vi "RvsTemp_Lakeshore_crh.vi"() -> ()   [LabVIEW 2017]
uses:
  sub_vis/ke26xx/Public/Channel.ctl
  sub_vis/ke26xx/KE26XX.lvlib
panel:
  in  "Units":i8(ring)=1 items=["Ohms"=1, "m-Ohms (1e-3)"=2, "u-Ohms (1e-6)"=3, ""=0]
  out "Neg. V (V)":dbl=1.0 format="%.;%#_g"
  out "Neg. I (A)":dbl=1.0 format="%.;%#_g"
  out "Pos. V (V)":dbl=1.0 format="%.;%#_g"
  out "Pos. I (A)":dbl=1.0 format="%.;%#_g"
  out "Node Out":string
  in  "Plot Scales":u16(ring) items=["Autoscale All", "Autoscale X", "Autoscale Y", "Manual Scale"]
  in  "Control Temp":bool=TRUE
  in  "Update":bool caption="Boolean"
  in  "Tab Control":enum32{"Configure", "Heater", "Auto"}(tab)
  in  "Curve Number (0)":dbl min=0.0 max=41.0 step=1.0
  in  "Sensor Type (0: Silicon Diode)":i8(ring) items=["Silicon Diode", "GaAIAS Diode", "100 Ohm Platinum/250", "100 Ohm Platinum/500", "1000 Ohm Platinum", "NTC RTD", "Thermo/25mV", "Thermo/50mV"]
  in  "Heater Range (0: Off)":u16(ring) items=["Off", "Low (0.5W)", "Med (5W)", "High (50W)"]
  in  "Manual Output (%)":dbl min=0.0 max=100.0 step=0.001 format="%.;%.3f"
  out "Heater Output":dbl(slide) scale=0.0..100.0
  in  "Loop (0: 1)":u16(ring) items=["1", "2"]
  in  "Rate (D)":dbl min=0.0 max=1000.0 step=0.1 format="%.;%.1f"
  in  "Reset (I)":dbl min=0.0 max=1000.0 step=0.1 format="%.;%.1f"
  in  "Gain (P)":dbl min=0.0 max=1000.0 step=0.1 format="%.;%.1f"
  in  "Ramp Rate\n(K/min)":dbl=0.1 min=0.0 max=100.0 step=0.1 format="%.1f"
  in  "Ramping \nOn/Off (F: Off)":bool
  in  "Setpoint (K)":dbl min=0.0 max=1000.0 step=0.1 format="%.;%.1f"
  in  "Control Mode (0: Manual PID)":u16(ring) items=["Manual PID", "Zone", "Open Loop", "AutoTune PID", "AutoTune PI", "AutoTune P"]
  out "temp vs time":cluster{"Y":dbl[], "Y":dbl[]}[](graph)
  out "Current (mA):":dbl=19.983 format="%.;%.4f"
  out "Voltage (mV):":dbl=19.983 format="%.;%.4f"
  in  "Limit (mA)":dbl=1.0 format="%.;%#_g"
  in  "Level (mV)":dbl=1.0 format="%.;%#_g"
  in  "Channel (A):":T1
  in  "VISA resource name":refnum<visa-resource-name>
  in  "Comments":string="comments here"
  in  "Y Max.":dbl min=0.0 max=1000.0 step=0.1 format="%.;%.1f"
  in  "Y Min.":dbl min=0.0 max=1000.0 step=0.1 format="%.;%.1f"
  in  "X Max.":dbl min=0.0 max=1000.0 step=0.1 format="%.;%.1f"
  in  "X Min.":dbl min=0.0 max=1000.0 step=0.1 format="%.;%.1f"
  in  "Reset":bool
  out "Resistance":dbl=19.983 format="%.;%_5f"
  in  "Log R":bool
  in  "Filename 2":string="07_YBCO_EOS_20K_outofplane_pumpon_5ps_"
  in  "Extension":string=".dat"
  in  "Filename":string="filename"
  in  "Path":string="C:\\path\\to\\data"
  in  "Save":bool caption="Boolean"
  in  "Log Temp":bool=TRUE
  in  "Lakeshore VISA session":refnum<visa-resource-name>="COM1"
  in  "Lakeshore Input (0: A)":u16(ring)=2 items=["A", "B", "ITC5035"]
  out "Temperature (K)":dbl=19.983 format="%.2f"
  in  "Stop":bool
  out "R vs T":cluster{"Y":dbl[], "Y":dbl[]}[](graph)
  # "Temperature Sensor"
  # "Set Filename and Path"
  # "Heater Control"
  # "Resistance Measurement"
  # "Written by Cassi Hunt, November 2012\n\nTemperature Control: LakeShore 331\nSourceMeter: Keithley 2635A"
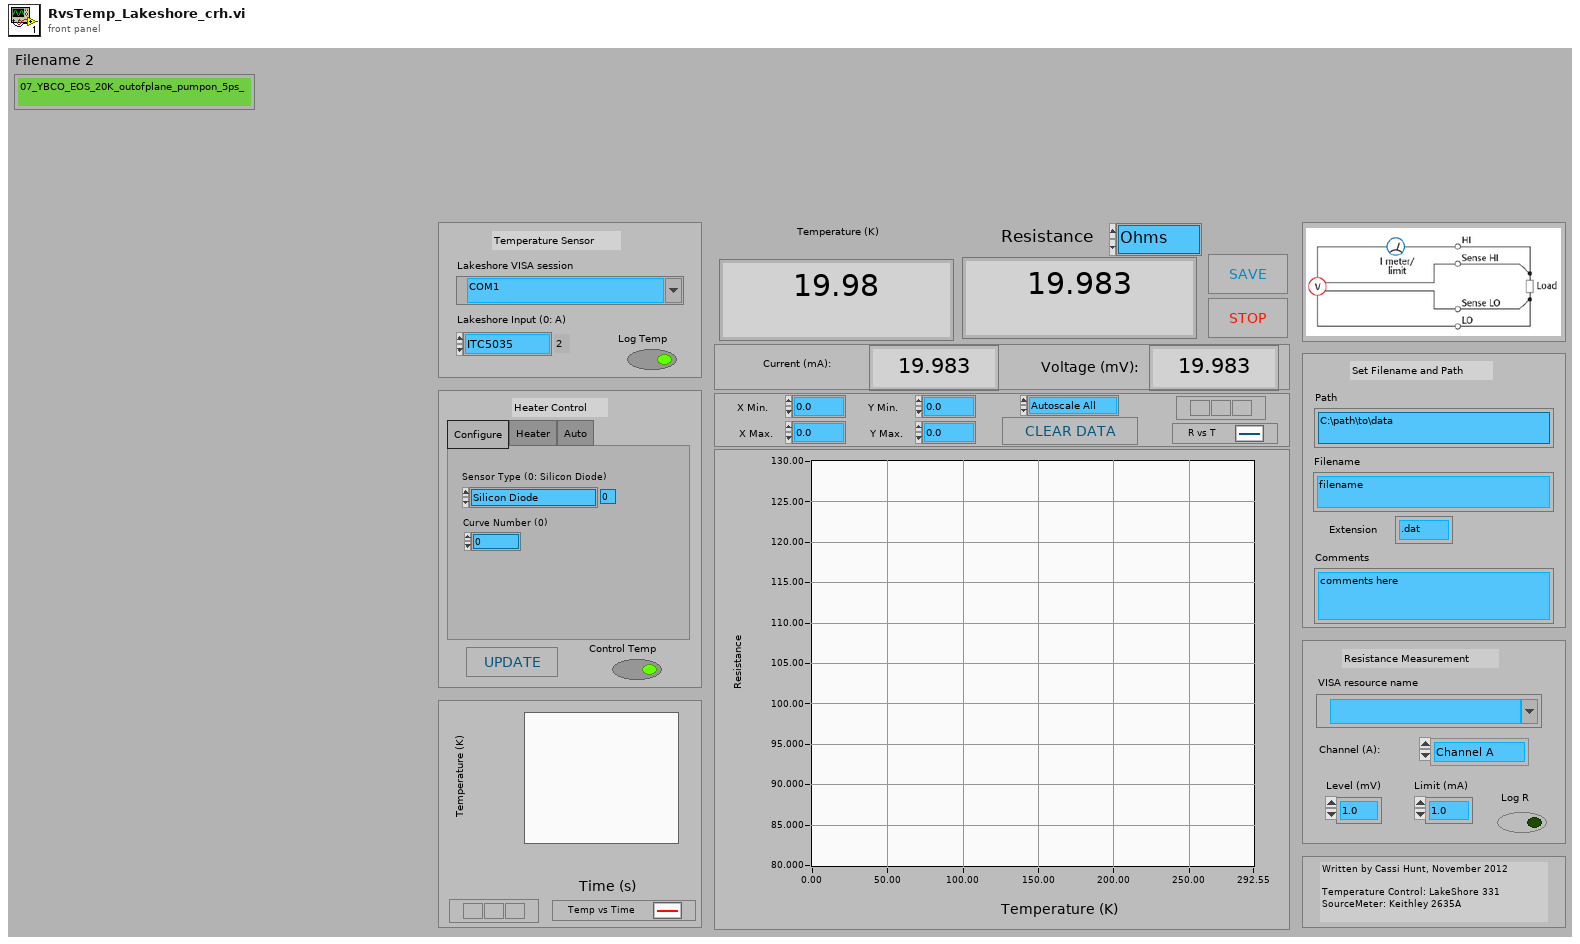
[diagram p1: front panel]
types:
  T1 = typedef "KE26XX.lvlib/Channel.ctl" = enum32{"Channel A", "Channel B"}
  T2 = enum32{"Current", "Voltage", "IV", "Resistance", "Power"}
  T3 = typedef "ke26xx.lvlib/Channel.ctl" = enum32{"Channel A", "Channel B"}
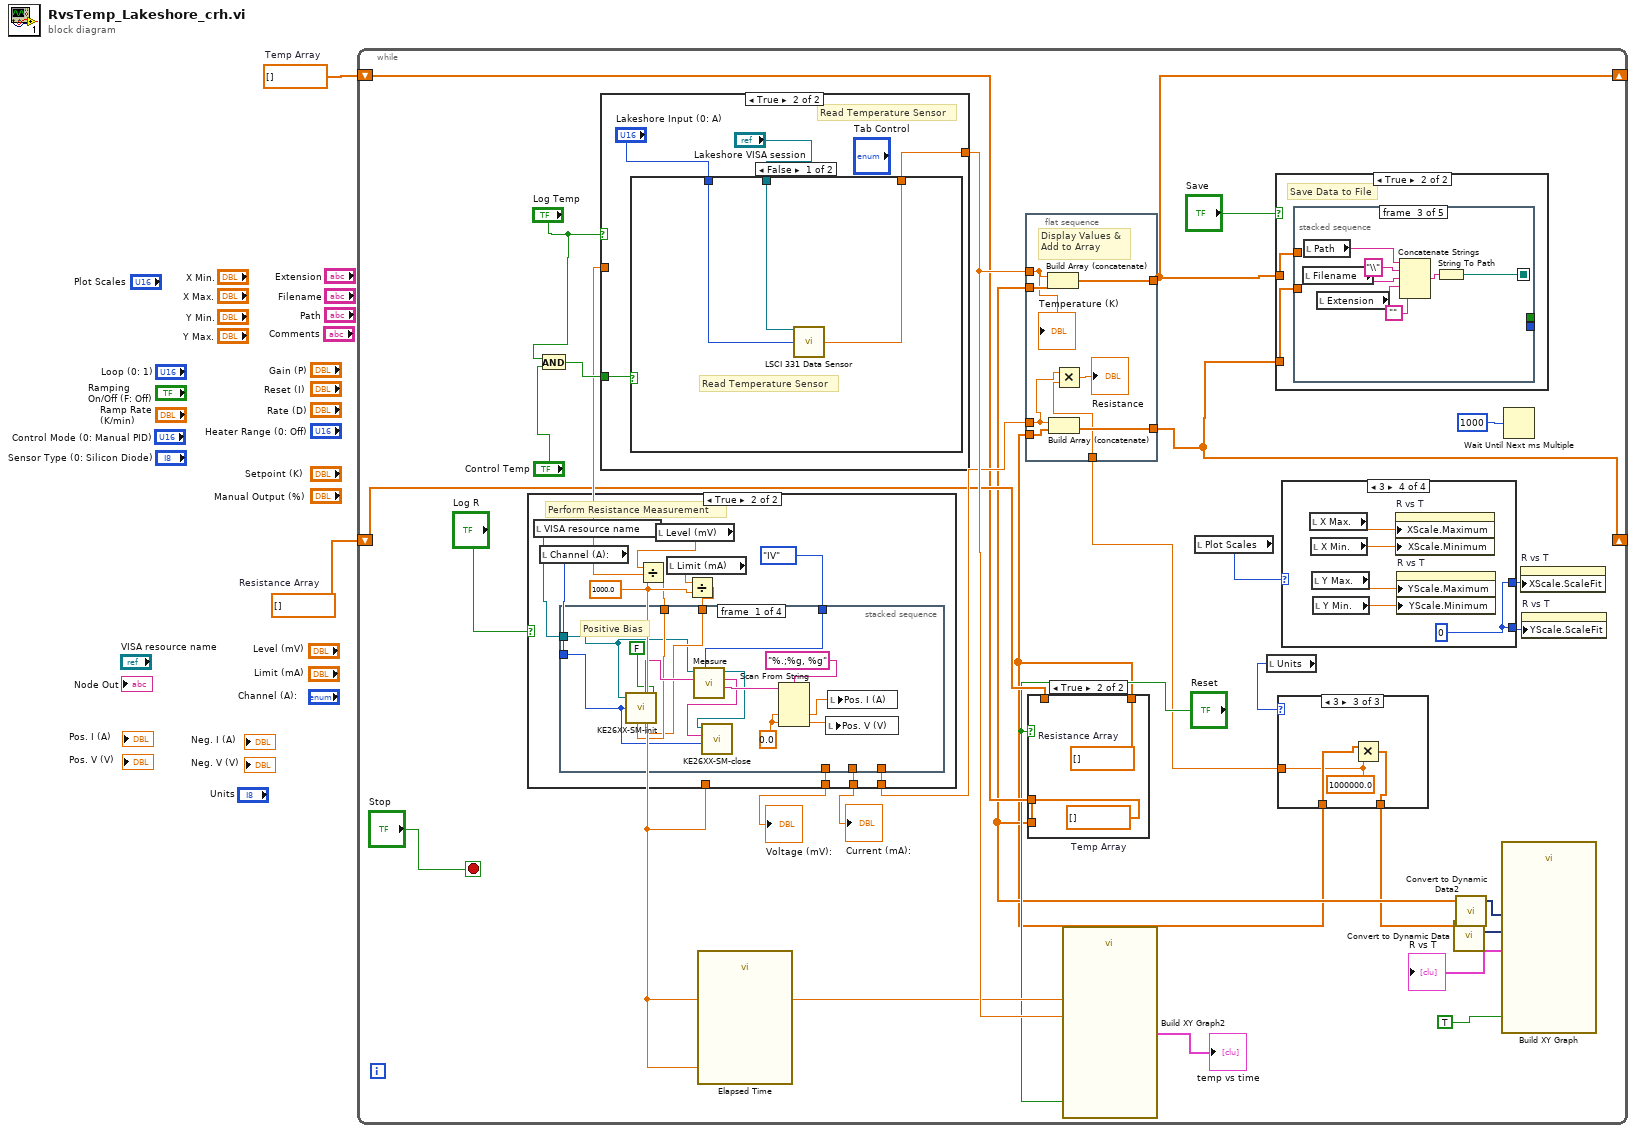
[diagram p0: block diagram]
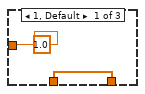
[diagram p2: hidden frame]
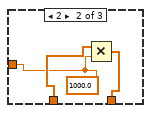
[diagram p3: hidden frame]
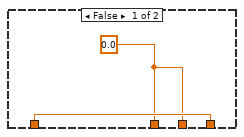
[diagram p5: hidden frame]
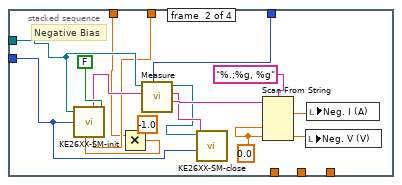
[diagram p6: hidden frame]
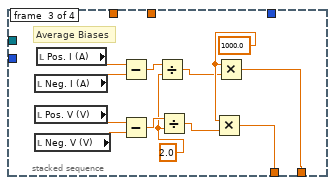
[diagram p7: hidden frame]
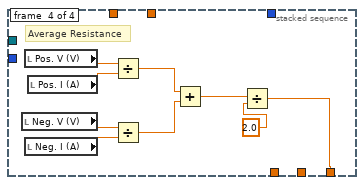
[diagram p8: hidden frame]
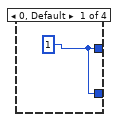
[diagram p9: hidden frame]
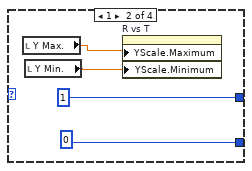
[diagram p10: hidden frame]
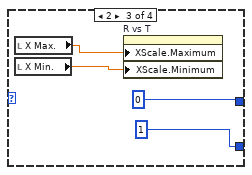
[diagram p11: hidden frame]
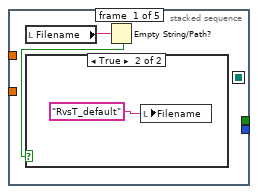
[diagram p13: hidden frame]
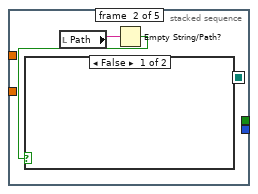
[diagram p15: hidden frame]
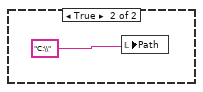
[diagram p16: hidden frame]
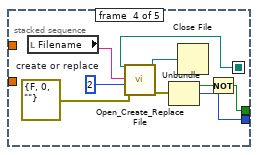
[diagram p17: hidden frame]
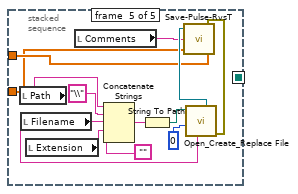
[diagram p18: hidden frame]
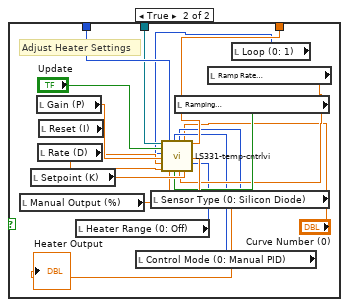
[diagram p20: hidden frame]
diagram:
  w1 = dbl[] []  # Resistance Array
  w2 = dbl[] []  # Temp Array
  n1 = while {
    shift-right: [w24] -> _
    shift-left: w2 -> [w13]
    shift-right: [w5] -> _
    shift-left: w1 -> [w14]
    stop <- "Stop" stop-if-true
    n2 = And(x="Log Temp", y="Control Temp") -> (x .and. y?=w27:bool)
    n3 = call "Elapsed Time"() -> ("Elapsed Time (s)"=w16:dbl)  [unwired: 12 in, 7 out]
    n4 = case shown="True" "Log R" {
      tunnel: [w46 w49] -> w19
      tunnel: [w45 w48] -> w18
      tunnel: [w45 w47] -> w17
      tunnel: w16 -> [w46 _]
      frame False {
        w45 = 0.0
      }
      frame True {
        w54 = 1000.0
        # "Perform Resistance Measurement"
        n5 = local read "VISA resource name"() -> (w57:refnum<visa-resource-name>)
        n6 = local read "Channel (A):"() -> (w56:T3)
        n7 = local read "Level (mV)"() -> (w51:dbl)
        n8 = Divide(x=w51, y=w54) -> (x/y=w50:dbl)
        n9 = local read "Limit (mA)"() -> (w53:dbl)
        n10 = Divide(x=w53, y=w54) -> (x/y=w52:dbl)
        n11 = stacked-sequence {
          tunnel: w57 -> [w64 w83 _ _]
          tunnel: w56 -> [w58 w73 _ _]
          tunnel: T2."IV" ("Measure Function (Current)") -> [w67 w81 _ _]
          tunnel: w52 -> [w65 w82 _ _]
          tunnel: w50 -> [w66 w76 _ _]
          tunnel: [_ _ _ w100] -> w49
          tunnel: [_ _ w89 _] -> w48
          tunnel: [_ _ w88 _] -> w47
          frame #0 {
            w70 = 0.0
            # "Positive Bias"
            n12 = call "KE26XX-SM-init.vi"("VISA resource name"=w64, "Channel (Channel A)"=w58, "Level"=w66, "Error Query (False)"=FALSE, "Limit"=w65) -> ("Node Out"=w68:string)  [unwired: 3 in, 1 out]
            n13 = call "Measure.vi"("Function (Current)"=w67, "Node In"=w68, "VISA resource name"=w64) -> ("Output"=w69:string, "Node Out"=w59:string, "VISA resource name out"=w60:refnum<visa-resource-name>)  [unwired: 4 in, 2 out]
            n14 = call "KE26XX-SM-close.vi"("Channel (Channel A)"=w58, "Node In"=w59, "VISA resource name"=w60) -> ()  [unwired: 8 in, 1 out]
            n15 = Scan From String(format string="%.;%g, %g", input string=w69, default 1=w70, default 2=w70) -> (output 1=w62:dbl, output 2=w61:dbl)  [unwired: 2 in, 3 out]
            n16 = local write "Pos. V (V)"(w61) -> ()
            n17 = local write "Pos. I (A)"(w62) -> ()
          }
          frame #1 {
            w84 = 0.0
            # "Negative Bias"
            n18 = Multiply(x=w76, y=-1.0) -> (x*y=w75:dbl)
            n19 = call "KE26XX-SM-init.vi"("VISA resource name"=w83, "Channel (Channel A)"=w73, "Level"=w75, "Error Query (False)"=FALSE, "Limit"=w82) -> ("Node Out"=w86:string)  [unwired: 3 in, 1 out]
            n20 = call "Measure.vi"("Function (Current)"=w81, "Node In"=w86, "VISA resource name"=w83) -> ("Output"=w85:string, "Node Out"=w74:string, "VISA resource name out"=w72:refnum<visa-resource-name>)  [unwired: 4 in, 2 out]
            n21 = call "KE26XX-SM-close.vi"("Channel (Channel A)"=w73, "Node In"=w74, "VISA resource name"=w72) -> ()  [unwired: 8 in, 1 out]
            n22 = Scan From String(format string="%.;%g, %g", input string=w85, default 1=w84, default 2=w84) -> (output 1=w79:dbl, output 2=w78:dbl)  [unwired: 2 in, 3 out]
            n23 = local write "Neg. V (V)"(w78) -> ()
            n24 = local write "Neg. I (A)"(w79) -> ()
          }
          frame #2 {
            w93 = 2.0
            w92 = 1000.0
            # "Average Biases"
            n25 = local read "Neg. I (A)"() -> (w98:dbl)
            n26 = local read "Pos. V (V)"() -> (w97:dbl)
            n27 = local read "Neg. V (V)"() -> (w96:dbl)
            n28 = local read "Pos. I (A)"() -> (w99:dbl)
            n29 = Subtract(x=w99, y=w98) -> (x-y=w94:dbl)
            n30 = Subtract(x=w97, y=w96) -> (x-y=w95:dbl)
            n31 = Divide(x=w94, y=w93) -> (x/y=w91:dbl)
            n32 = Divide(x=w95, y=w93) -> (x/y=w90:dbl)
            n33 = Multiply(x=w92, y=w90) -> (x*y=w88:dbl)
            n34 = Multiply(x=w92, y=w91) -> (x*y=w89:dbl)
          }
          frame #3 {
            # "Average Resistance"
            n35 = local read "Neg. V (V)"() -> (w106:dbl)
            n36 = local read "Pos. V (V)"() -> (w108:dbl)
            n37 = local read "Neg. I (A)"() -> (w105:dbl)
            n38 = local read "Pos. I (A)"() -> (w107:dbl)
            n39 = Divide(x=w108, y=w107) -> (x/y=w104:dbl)
            n40 = Divide(x=w106, y=w105) -> (x/y=w103:dbl)
            n41 = Add(x=w104, y=w103) -> (x+y=w102:dbl)
            n42 = Divide(x=w102, y=2.0) -> (x/y=w100:dbl)
          }
        }
      }
    }
    "Voltage (mV):" <- w17
    "Current (mA):" <- w18
    n43 = case shown="True" "Log Temp" {
      tunnel: [w168 w169] -> w25
      tunnel: w16 -> [w168 _]
      tunnel: w27 -> [_ w172]
      frame False {
      }
      frame True {
        # "Read Temperature Sensor"
        n44 = case shown="False" w172 {
          tunnel: "Lakeshore Input (0: A)" -> [w173 w192]
          tunnel: "Lakeshore VISA session" -> [w174 w191]
          tunnel: [w175 w183] -> w169
          frame False {
            # "Read Temperature Sensor"
            n45 = call "LSCI 331 Data Sensor.vi"("VISA session"=w174, "Input (0: A)"=w173) -> ("Kelvin Reading"=w175:dbl)  [unwired: 1 in, 12 out]
          }
          frame True {
            # "Adjust Heater Settings"
            n46 = local read "Manual Output (%)"() -> (w185:dbl)
            n47 = local read "Setpoint (K)"() -> (w186:dbl)
            n48 = local read "Gain (P)"() -> (w189:dbl)
            n49 = local read "Rate (D)"() -> (w187:dbl)
            n50 = local read "Reset (I)"() -> (w188:dbl)
            n51 = local read "Heater Range (0: Off)"() -> (w179:u16)
            n52 = local read "Control Mode (0: Manual PID)"() -> (w178:u16)
            n53 = local read "Sensor Type (0: Silicon Diode)"() -> (w177:i8)
            n54 = local read "Ramping \nOn/Off (F: Off)"() -> (w182:bool)
            n55 = local read "Ramp Rate\n(K/min)"() -> (w180:dbl)
            n56 = local read "Loop (0: 1)"() -> (w181:u16)
            n57 = call "LS331-temp-cntrlvi.vi"("VISA resource name"=w191, "Configure (False)"="Update", "Loop (0: 1)"=w181, "Gain (P) (0.0)"=w189, "Reset (I) (0.0)"=w188, "Rate (D) (0)"=w187, "Input (0: A)"=w192, "Control Mode (0: Manual PID)"=w178, "Ramping On/Off (F: Off)"=w182, "Sensor Type (0: Silicon Diode)"=w177, "Rate Value (0.1)"=w180, "Curve Number (0)"="Curve Number (0)", "Setpoint (0.0000)"=w186, "Manual Output (0.000)"=w185, "Heater Range (0: Off)"=w179) -> ("Loop 1\nHeater Output"=→"Heater Output":dbl, "Kelvin Reading"=w183:dbl)  [unwired: 1 in, 2 out]
          }
        }
      }
    }
    n58 = flat-sequence {
      tunnel: w9 -> [w129]
      tunnel: [w130] -> w24
      tunnel: w25 -> [w126]
      tunnel: w19 -> [w125]
      tunnel: w7 -> [w127]
      tunnel: [w128] -> w5
      tunnel: w4 -> [w123]
      frame #0 {
        # "Display Values &\nAdd to Array"
        n59 = Build Array (concatenate)(w126, w129) -> (w130:dbl[])
        n60 = Build Array (concatenate)(w125, w127) -> (w128:dbl[])
        n61 = Multiply(x=w125, y=w123) -> (x*y=→"Resistance":dbl)
        "Temperature (K)" <- w126
      }
    }
    n62 = case shown="True" "Reset" {
      tunnel: [w42 w44] -> w7
      tunnel: w14 -> [w42 _]
      tunnel: [w41 w43] -> w9
      tunnel: w13 -> [w41 _]
      frame False {
      }
      frame True {
        w43 = dbl[] []  # Temp Array
        w44 = dbl[] []  # Resistance Array
      }
    }
    n63 = call "Build XY Graph2"("Reset"="Reset", "Y Input"=w25, "X Input"=w16) -> ("XY Graph"=→"temp vs time":cluster{"Y":dbl[], "Y":dbl[]}[])  [unwired: 2 in, 6 out]
    n64 = local read "Plot Scales"() -> (w23:u16)
    n65 = local read "Units"() -> (w11:i8)
    n66 = case shown="True" "Save" {
      tunnel: w24 -> [_ w132]
      tunnel: w5 -> [_ w131]
      frame False {
      }
      frame True {
        # "Save Data to File"
        n67 = stacked-sequence {
          seq-local: [_ _ w143 _ _] -> [_ _ _ w148 _]
          tunnel: [_ _ _ w149 _] -> _
          tunnel: [_ _ _ w147 _] -> _
          tunnel: w132 -> [_ _ _ _ w157]
          tunnel: w131 -> [_ _ _ _ w156]
          frame #0 {
            n68 = local read "Filename"() -> (w134:string)
            n69 = Empty String/Path?(string/path=w134) -> (empty?=w133:bool)
            n70 = case shown="True" w133 {
              frame False {
              }
              frame True {
                n71 = local write "Filename"("RvsT_default") -> ()
              }
            }
          }
          frame #1 {
            n72 = local read "Path"() -> (w137:string)
            n73 = Empty String/Path?(string/path=w137) -> (empty?=w136:bool)
            n74 = case shown="False" w136 {
              frame False {
              }
              frame True {
                n75 = local write "Path"("C:\\") -> ()
              }
            }
          }
          frame #2 {
            n76 = local read "Filename"() -> (w139:string)
            n77 = local read "Path"() -> (w142:string)
            n78 = local read "Extension"() -> (w140:string)
            n79 = Concatenate Strings(w142, "\\" ("Substring"), w139, w140, "") -> (w144:string)
            n80 = String To Path(string=w144) -> (path=w143:path)
          }
          frame #3 {
            w151 = i16 2  # create or replace
            n81 = local read "Filename"() -> (w146:string)
            n82 = call <vilib>:"Open_Create_Replace File.vi"("default name"=w146, "error in (no error)"=errorcluster {"status"=FALSE, "code"=0, "source"=""}, "function (open:0)"=w151, "file path"=w148) -> ("error out"=w153:errorcluster, "refnum"=w152:refnum<file>)  [unwired: 2 in, 4 out]
            n83 = Unbundle(w153) -> ("status"=w150:bool, "code"=w147:i32)  [unwired: 1 out]
            n84 = Close File(refnum=w152) -> ()  [unwired: 1 in, 2 out]
            n85 = Not(x=w150) -> (.not. x?=w149:bool)
          }
          frame #4 {
            n86 = local read "Path"() -> (w158:string)
            n87 = local read "Filename"() -> (w164:string)
            n88 = local read "Extension"() -> (w160:string)
            n89 = local read "Comments"() -> (w155:string)
            n90 = Concatenate Strings(w158, "\\" ("Substring"), w164, w160, "") -> (w161:string)
            n91 = String To Path(string=w161) -> (path=w162:path)
            n92 = call <vilib>:"Open_Create_Replace File.vi"("default name"=w164, "function (open:0)"=i16 0 ("create or replace"), "file path"=w162) -> ("error out"=w166:errorcluster, "refnum"=w167:refnum<file>)  [unwired: 3 in, 4 out]
            n93 = call "Save-Pulse-RvsT.vi"("X-Values"=w157, "error in"=w166, "Y-Values"=w156, "comment"=w155, "refnum"=w167) -> ()  [unwired: 1 out]
          }
        }
      }
    }
    n94 = case shown="3" w11 {
      tunnel: w7 -> [w34 w37 w40]
      tunnel: [w34 w35 w39] -> w6
      tunnel: [1.0 w36 w38] -> w4
      frame 1, Default {
      }
      frame 2 {
        w36 = 1000.0
        n95 = Multiply(x=w37, y=w36) -> (x*y=w35:dbl[])
      }
      frame 3 {
        w38 = 1000000.0
        n96 = Multiply(x=w40, y=w38) -> (x*y=w39:dbl[])
      }
    }
    n97 = case shown="3" w23 {
      tunnel: [w109 1 0 w122] -> w21
      tunnel: [w109 0 1 w122] -> w22
      frame 0, Default {
        w109 = 1
      }
      frame 1 {
        n98 = local read "Y Max."() -> (w112:dbl)
        n99 = local read "Y Min."() -> (w113:dbl)
        n100 = property on="R vs T" class="XYGraph (strict)"("YScale.Maximum"=w112, "YScale.Minimum"=w113) -> ()  [unwired: 2 in, 2 out]
      }
      frame 2 {
        n101 = local read "X Max."() -> (w117:dbl)
        n102 = local read "X Min."() -> (w116:dbl)
        n103 = property on="R vs T" class="XYGraph (strict)"("XScale.Maximum"=w117, "XScale.Minimum"=w116) -> ()  [unwired: 2 in, 2 out]
      }
      frame 3 {
        w122 = 0
        n104 = local read "X Max."() -> (w121:dbl)
        n105 = local read "X Min."() -> (w120:dbl)
        n106 = local read "Y Max."() -> (w119:dbl)
        n107 = local read "Y Min."() -> (w118:dbl)
        n108 = property on="R vs T" class="XYGraph (strict)"("XScale.Maximum"=w121, "XScale.Minimum"=w120) -> ()  [unwired: 2 in, 2 out]
        n109 = property on="R vs T" class="XYGraph (strict)"("YScale.Maximum"=w119, "YScale.Minimum"=w118) -> ()  [unwired: 2 in, 2 out]
      }
    }
    n110 = call "Convert to Dynamic Data"("Array"=w6) -> ("Dynamic Data Type"=w10:dynamicdata)  [unwired: 3 in]
    n111 = call "Convert to Dynamic Data2"("Array"=w9) -> ("Dynamic Data Type"=w8:dynamicdata)  [unwired: 3 in]
    n112 = call "Build XY Graph"("Reset"=TRUE, "Y Input"=w10, "X Input"=w8) -> ("XY Graph"=→"R vs T":cluster{"Y":dbl[], "Y":dbl[]}[])  [unwired: 2 in, 6 out]
    n113 = Wait Until Next ms Multiple(millisecond multiple=u32 1000) -> ()  [unwired: 1 out]
    n114 = property on="R vs T" class="XYGraph (strict)"("XScale.ScaleFit"=w21) -> ()  [unwired: 2 in, 2 out]
    n115 = property on="R vs T" class="XYGraph (strict)"("YScale.ScaleFit"=w22) -> ()  [unwired: 2 in, 2 out]
  }
